vi "A13rowin.vi"(11 "Basic Size":dbl) -> (3 "Row":dbl)   [LabVIEW 2023]
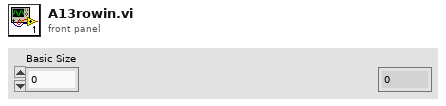
[diagram p1: front panel]
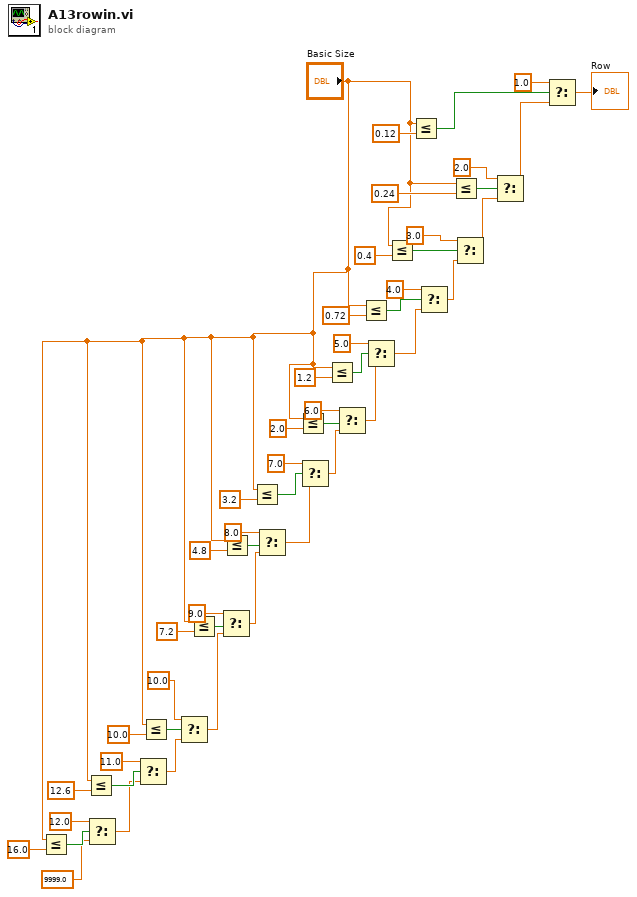
[diagram p0: block diagram]
diagram:
  n1 = Less Or Equal?(x="Basic Size", y=16.0) -> (x <= y?=w5:bool)
  n2 = Less Or Equal?(x="Basic Size", y=12.6) -> (x <= y?=w9:bool)
  n3 = Select(t=12.0, s=w5, f=9999.0) -> (s? t:f=w7:dbl)
  n4 = Select(t=11.0, s=w9, f=w7) -> (s? t:f=w11:dbl)
  n5 = Less Or Equal?(x="Basic Size", y=10.0) -> (x <= y?=w13:bool)
  n6 = Select(t=10.0, s=w13, f=w11) -> (s? t:f=w15:dbl)
  n7 = Less Or Equal?(x="Basic Size", y=7.2) -> (x <= y?=w17:bool)
  n8 = Select(t=9.0, s=w17, f=w15) -> (s? t:f=w19:dbl)
  n9 = Less Or Equal?(x="Basic Size", y=4.8) -> (x <= y?=w21:bool)
  n10 = Less Or Equal?(x="Basic Size", y=3.2) -> (x <= y?=w25:bool)
  n11 = Select(t=8.0, s=w21, f=w19) -> (s? t:f=w23:dbl)
  n12 = Less Or Equal?(x="Basic Size", y=2.0) -> (x <= y?=w29:bool)
  n13 = Select(t=7.0, s=w25, f=w23) -> (s? t:f=w27:dbl)
  n14 = Less Or Equal?(x="Basic Size", y=1.2) -> (x <= y?=w33:bool)
  n15 = Select(t=6.0, s=w29, f=w27) -> (s? t:f=w31:dbl)
  n16 = Less Or Equal?(x="Basic Size", y=0.72) -> (x <= y?=w37:bool)
  n17 = Select(t=5.0, s=w33, f=w31) -> (s? t:f=w35:dbl)
  n18 = Less Or Equal?(x="Basic Size", y=0.4) -> (x <= y?=w41:bool)
  n19 = Less Or Equal?(x="Basic Size", y=0.12) -> (x <= y?=w50:bool)
  n20 = Select(t=4.0, s=w37, f=w35) -> (s? t:f=w39:dbl)
  n21 = Less Or Equal?(x="Basic Size", y=0.24) -> (x <= y?=w46:bool)
  n22 = Select(t=3.0, s=w41, f=w39) -> (s? t:f=w43:dbl)
  n23 = Select(t=2.0, s=w46, f=w43) -> (s? t:f=w48:dbl)
  n24 = Select(t=1.0, s=w50, f=w48) -> (s? t:f=→"Row":dbl)
